vi "SubDaqProcess.vi"(7 "MainQueueIN":refnum<queue>, 8 "error in (no error)":errorcluster, 9 "SubDaqCommand":T1, 10 "SubQueueIN":refnum<queue>, 11 "Data Value Reference IN":refnum<data-value>) -> (0 "error out":errorcluster, 3 "Data Value Reference out":refnum<data-value>)   [LabVIEW 2013]
uses:
  Control/SystemData.ctl
  Control/SignalType.ctl
  Control/SystemCommand.ctl
  Control/SubDaqCommand.ctl
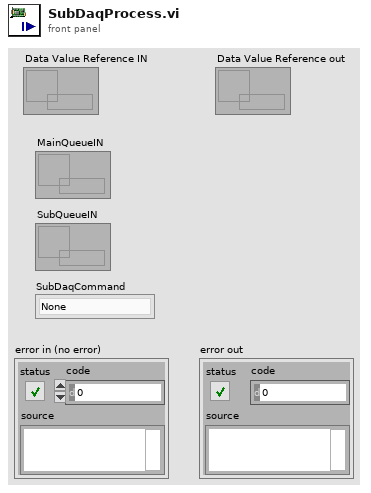
[diagram p1: front panel]
types:
  T1 = typedef "SubDaqCommand.ctl" = enum16{"None", "Init", "Work", "Stop", "Close"}
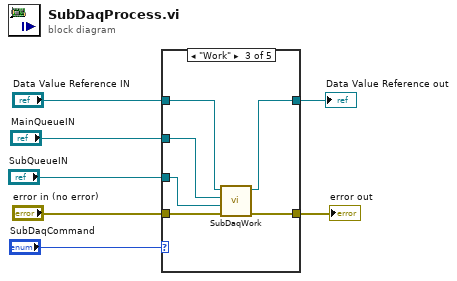
[diagram p0: block diagram]
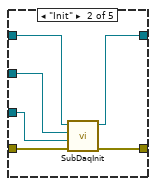
[diagram p3: hidden frame]
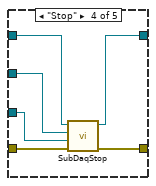
[diagram p4: hidden frame]
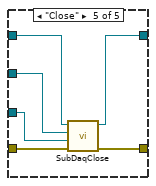
[diagram p5: hidden frame]
diagram:
  n1 = case shown="\"Work\"" "SubDaqCommand" {
    tunnel: "Data Value Reference IN" -> [w9 w13 w19 w25 w31]
    tunnel: [w9 w12 w18 w24 w30] -> w6
    tunnel: "error in (no error)" -> [w8 w15 w21 w27 w33]
    tunnel: [w8 w14 w20 w26 w32] -> w7
    tunnel: "MainQueueIN" -> [_ w11 w17 w23 w29]
    tunnel: "SubQueueIN" -> [_ w10 w16 w22 w28]
    frame Default {
    }
    frame "Init" {
      n2 = call "SubDaqInit.vi"("error in (no error)"=w15, "SubQueueIN"=w10, "MainQueueIN"=w11, "Data Value Reference IN"=w13) -> ("error out"=w14:errorcluster, "Data Value Reference out"=w12:refnum<data-value>)  [unwired: 6 in]
    }
    frame "Work" {
      n3 = call "SubDaqWork.vi"("error in (no error)"=w21, "SubQueueIN"=w16, "MainQueueIN"=w17, "Data Value Reference IN"=w19) -> ("error out"=w20:errorcluster, "Data Value Reference out"=w18:refnum<data-value>)  [unwired: 6 in]
    }
    frame "Stop" {
      n4 = call "SubDaqStop.vi"("error in (no error)"=w27, "SubQueueIN"=w22, "MainQueueIN"=w23, "Data Value Reference IN"=w25) -> ("error out"=w26:errorcluster, "Data Value Reference out"=w24:refnum<data-value>)  [unwired: 6 in]
    }
    frame "Close" {
      n5 = call "SubDaqClose.vi"("error in (no error)"=w33, "SubQueueIN"=w28, "MainQueueIN"=w29, "Data Value Reference IN"=w31) -> ("error out"=w32:errorcluster, "Data Value Reference out"=w30:refnum<data-value>)  [unwired: 6 in]
    }
  }
  "error out" <- w7
  "Data Value Reference out" <- w6
